vi "Disconnect.vi"(8 "error in (no error)":errorcluster, 11 "TCP Comm":T1) -> (0 "error out":errorcluster)   [LabVIEW 2020, in "TinyTCP.lvlib"]
uses:
  TinyTCP.lvlib
  Instance.ctl
  Ref Data.ctl
  State.ctl
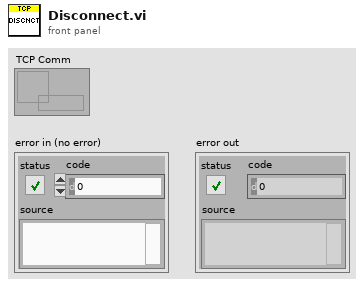
[diagram p1: front panel]
types:
  T1 = typedef "TinyTCP.lvlib/Instance.ctl" = refnum<data-value>
  T2 = typedef "TinyTCP.lvlib/State.ctl" = enum16{"Idle", "Starting", "Connecting", "Connected", "Disconnecting", "Stopped"}
  T3 = typedef "TinyTCP.lvlib/Ref Data.ctl" = cluster{"TCP":refnum<k5>, "State":T2, "Server":bool, "Host":string, "Port":u16, "Listener":refnum<k5>, "Start":bool, "Disconnect":bool, "TCP Valid":bool, "TLS Enabled":bool, "Immutable TLS":refnum<k36>, "Certificate DN":string, "local-port":u16}
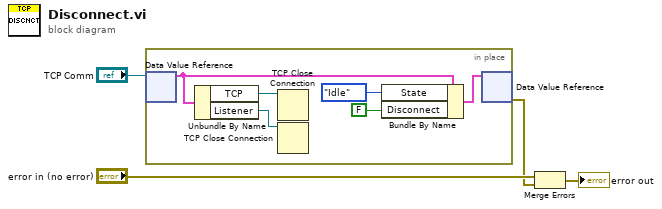
[diagram p0: block diagram]
diagram:
  n1 = in-place {
    n2 = in-place-dvr #1("TCP Comm") -> (w10:T3)  [unwired: 1 out]
    n3 = Unbundle By Name(w10) -> ("TCP"=w7:refnum<k5>, "Listener"=w8:refnum<k5>)
    n4 = TCP Close Connection(connection ID=w7) -> ()  [unwired: 2 in, 2 out]
    n5 = TCP Close Connection(connection ID=w8) -> ()  [unwired: 2 in, 2 out]
    n6 = Bundle By Name(cluster=w10, "State"=State."Idle", "Disconnect"=FALSE) -> (w9:T3)
    n7 = in-place-dvr #1(w9) -> (w1:errorcluster)  [unwired: 1 out]
  }
  n8 = Merge Errors("error in (no error)", w1) -> (→"error out":errorcluster)
